vi "Flash_replace.vi"(7 "DUT":string, 8 "error in":errorcluster, 10 "Array":string[](array[string])=["COM50", "D:\\Users\\A. Halstesd Evander\\Documents\\DTU_Manual_Flash\\Info\\Configuration\\RX01_DTU_N58_Application_0_0_10.pac", "E:\\Users\\A. Halstesd Evander\\Downloads\\RESEARCHDOWNLOAD_R22.19.1701\\RESEARCHDOWNLOAD_R22.19.1701\\Bin\\CmdDloader.exe", "F:\\Users\\A. Halstesd Evander\\Downloads\\RESEARCHDOWNLOAD_R22.19.1701\\RESEARCHDOWNLOAD_R22.19.1701\\Bin\\result.txt"], 11 "file path (use dialog)":path) -> (0 "error out":errorcluster)   [LabVIEW 2024, in "Neoway_flashing.lvlib"]
uses:
  Neoway_flashing.lvlib
  Launcher/Launcher_DTU.lvlib
panel:
  out "String":string
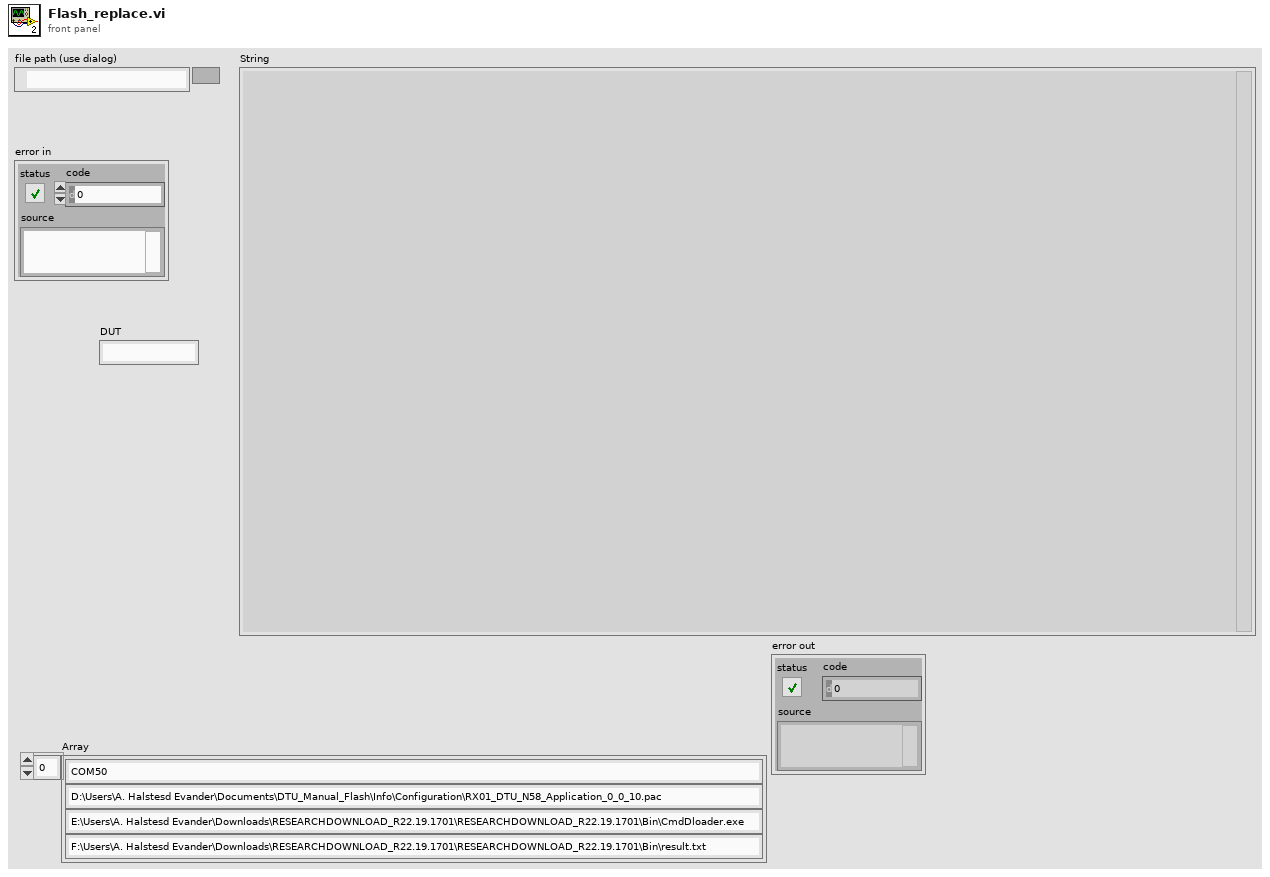
[diagram p1: front panel]
types:
  T1 = enum16{"Read", "Write", "All_sections", "All_values", "Remove key&section"}
  T2 = enum16{"open", "replace", "create", "open or create", "replace or create", "replace or create with confirmation"}
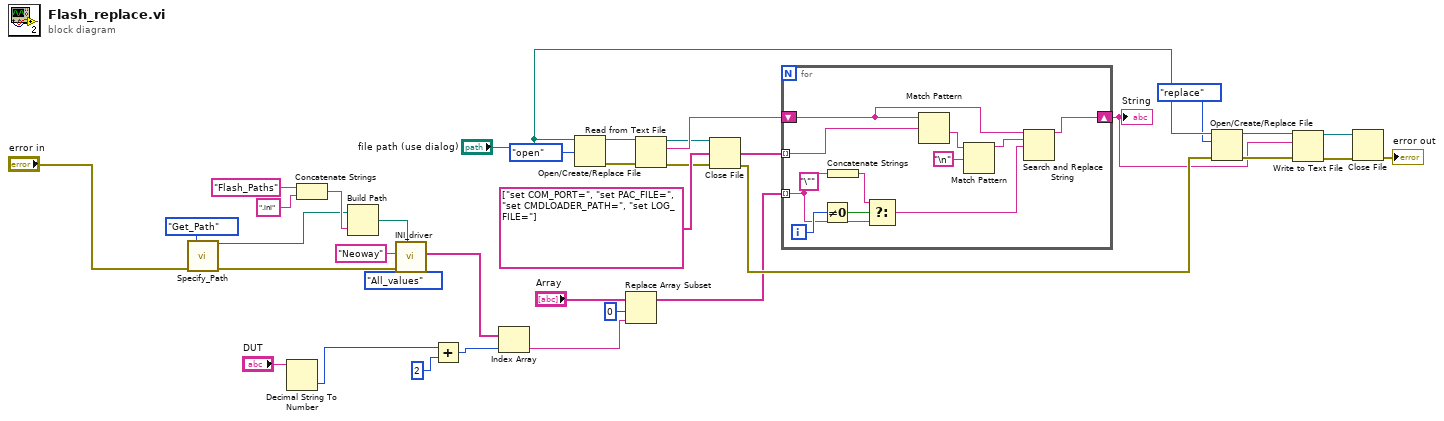
[diagram p0: block diagram]
diagram:
  n1 = call "Specify_Path.vi"("Path_Enum"=enum16{"Find_Path", "Get_Path"}."Get_Path", "error in (no error)"="error in") -> ("Configurations"=w10:path, "error out"=w14:errorcluster)  [unwired: 6 in, 6 out]
  n2 = Decimal String To Number(string="DUT") -> (number=w1:i32)  [unwired: 2 in, 1 out]
  n3 = Concatenate Strings("Flash_Paths" ("string"), ".ini" ("string")) -> (w16:string)
  n4 = Build Path(base path=w10, name or relative path=w16) -> (appended path=w15:path)
  n5 = call "INI_driver.vi"("Enum"=T1."All_values", "instrument file path"=w15, "error in (no error)"=w14, "Section"="Neoway") -> ("Values out"=w8:string[])  [unwired: 4 in, 3 out]
  n6 = Add(x=w1, y=2) -> (x+y=w3:i32)
  n7 = Index Array(array=w8, index=w3) -> (element=w5:string)
  n8 = Open/Create/Replace File(file path (use dialog)="file path (use dialog)", operation (0:open)=T2."open") -> (refnum out=w33:refnum<file>, error out=w34:errorcluster)  [unwired: 4 in, 1 out]
  n9 = Replace Array Subset(array="Array", new element=w5, index=0) -> (w7:string[])
  n10 = Read from Text File(file (use dialog)=w33, error in=w34) -> (refnum out=w28:refnum<file>, text=w31:string, error out=w29:errorcluster)  [unwired: 2 in, 1 out]
  n11 = Close File(refnum=w28, error in=w29) -> (error out=w25:errorcluster)  [unwired: 1 out]
  n12 = for {
    tunnel: string[] ["set COM_PORT=", "set PAC_FILE=", "set CMDLOADER_PATH=", "set LOG_FILE="] -> [w46] mode=indexing
    shift-right: [w39] -> w20
    shift-left: w31 -> [w45]
    tunnel: w7 -> [w41] mode=indexing
    i -> [w43]
    (unwired) "\"" ("string")
    n13 = Not Equal To 0?(x=w43) -> (x != 0?=w44:bool)
    n14 = Concatenate Strings(w41) -> (w42:string)
    n15 = Select(t=w42, s=w44, f=w41) -> (s? t:f=w40:string)
    n16 = Match Pattern(string=w45, regular expression=w46) -> (after substring=w38:string)  [unwired: 1 in, 3 out]
    n17 = Match Pattern(string=w38, regular expression="\n") -> (before substring=w36:string)  [unwired: 1 in, 3 out]
    n18 = Search and Replace String(input string=w45, search string=w36, replace string=w40) -> (result string=w39:string)  [unwired: 5 in, 3 out]
  }
  "String" <- w20
  n19 = Open/Create/Replace File(file path (use dialog)="file path (use dialog)", error in=w25, operation (0:open)=T2."replace") -> (refnum out=w24:refnum<file>, error out=w23:errorcluster)  [unwired: 3 in, 1 out]
  n20 = Write to Text File(file (use dialog)=w24, text=w20, error in=w23) -> (refnum out=w21:refnum<file>, error out=w22:errorcluster)  [unwired: 1 in, 1 out]
  n21 = Close File(refnum=w21, error in=w22) -> (error out=→"error out":errorcluster)  [unwired: 1 out]
